vi "PCO_GetCameraDescription_Intensified.vi"(8 "error in (no error)":errorcluster {"code" format="%x"}, 11 "ph":u64) -> (0 "error out":errorcluster {"code" format="%x"}, 1 "strDescription":T1 {"dwFlagsIntensifiedDESC" format="%x"}, 2 "ErrorMessage":i32 format="%x", 3 "ph out":u64)   [LabVIEW 2020, in "SDK.lvlib" / "SpecialCommandsDicam.lvlib"]
doc: "<b>Description:</b>\nAny of the available sensor and camera specific description can be queried. With input parameter wType the returned description structure can be selected. PCO_DescriptionEx is a generic structure which has to be casted to/from the queried structure. The wSize parameter has to be filled with the correct value for the requested structure. This function was introduced due to the size limitation of the standard camera descriptor and the need for describing additional features.\n\n<b>Supported camera type:</b>\nAll cameras\n\n<b>Descriptor dependency:</b>\ndwGeneralCapsDESC1: ENHANCED_DESCRIPTOR_2"
uses:
  SpecialCommandsDicam.lvlib
  Structures.lvlib
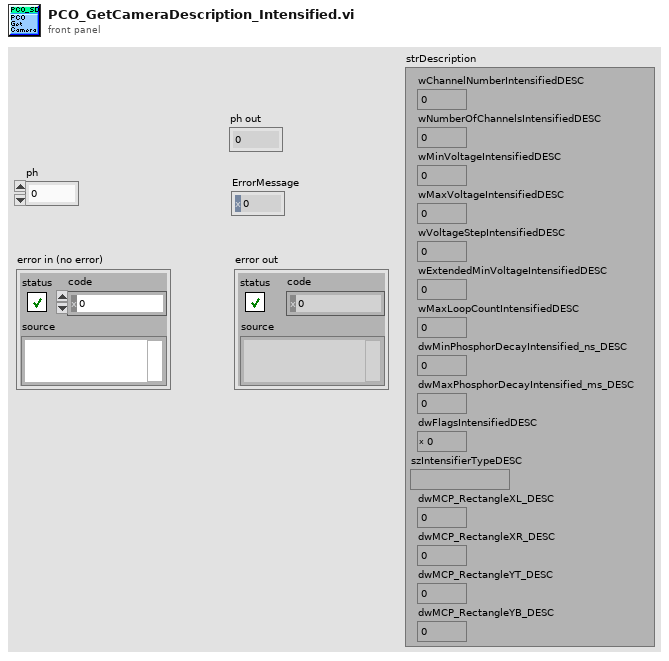
[diagram p1: front panel]
types:
  T1 = cluster{"wChannelNumberIntensifiedDESC":u16, "wNumberOfChannelsIntensifiedDESC":u16, "wMinVoltageIntensifiedDESC":u16, "wMaxVoltageIntensifiedDESC":u16, "wVoltageStepIntensifiedDESC":u16, "wExtendedMinVoltageIntensifiedDESC":u16, "wMaxLoopCountIntensifiedDESC":u16, "dwMinPhosphorDecayIntensified_ns_DESC":u32, "dwMaxPhosphorDecayIntensified_ms_DESC":u32, "dwFlagsIntensifiedDESC":u32, "szIntensifierTypeDESC":string, "dwMCP_RectangleXL_DESC":u32, "dwMCP_RectangleXR_DESC":u32, "dwMCP_RectangleYT_DESC":u32, "dwMCP_RectangleYB_DESC":u32}
  T2 = cluster{"wSize":u16, "wChannelNumberIntensifiedDESC":u16, "wNumberOfChannelsIntensifiedDESC":u16, "wMinVoltageIntensifiedDESC":u16, "wMaxVoltageIntensifiedDESC":u16, "wVoltageStepIntensifiedDESC":u16, "wExtendedMinVoltageIntensifiedDESC":u16, "wMaxLoopCountIntensifiedDESC":u16, "dwMinPhosphorDecayIntensified_ns_DESC":u32, "dwMaxPhosphorDecayIntensified_ms_DESC":u32, "dwFlagsIntensifiedDESC":u32, "szIntensifierTypeDESC":cluster{u8, u8, u8, u8, u8, u8, u8, u8, u8, u8, u8, u8, u8, u8, u8, u8, u8, u8, u8, u8, u8, u8, u8, u8}, "dwMCP_RectangleXL_DESC":u32, "dwMCP_RectangleXR_DESC":u32, "dwMCP_RectangleYT_DESC":u32, "dwMCP_RectangleYB_DESC":u32, "ZZdwDummy":cluster{u32, u32, u32, u32, u32, u32, u32, u32, u32, u32, u32, u32, u32, u32, u32, u32, u32, u32, u32, u32, u32, u32, u32}}
  T3 = cluster{u8, u8, u8, u8, u8, u8, u8, u8, u8, u8, u8, u8, u8, u8, u8, u8, u8, u8, u8, u8, u8, u8, u8, u8}
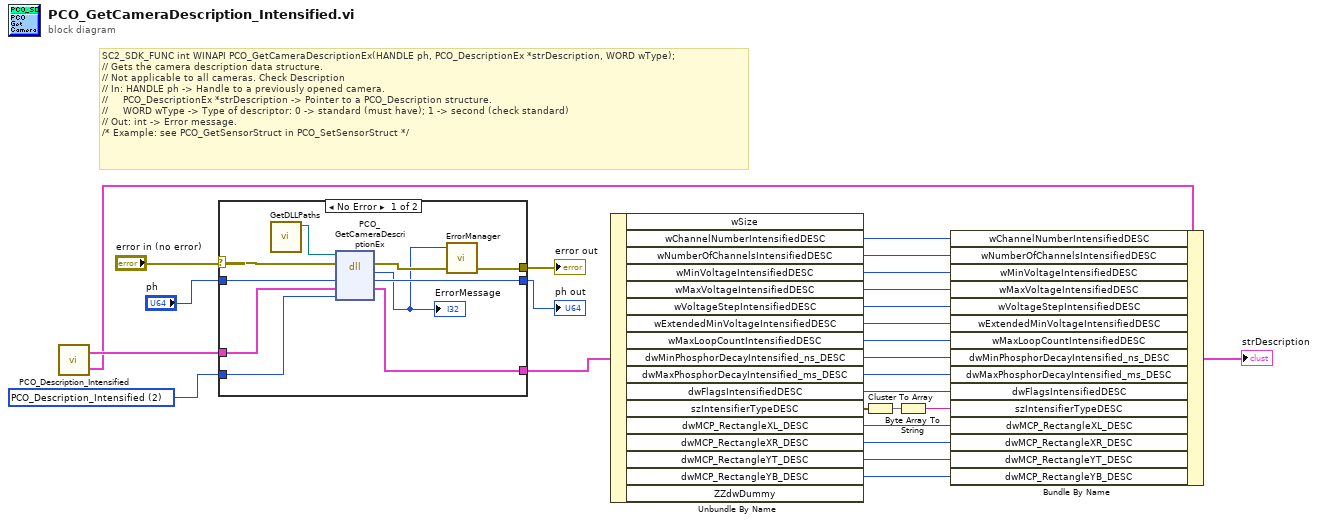
[diagram p0: block diagram]
diagram:
  w21 = u16 2 items=["PCO_Description", "PCO_Description2", "PCO_Description_Intensified"] ("wType")
  # "SC2_SDK_FUNC int WINAPI PCO_GetCameraDescriptionEx(HANDLE ph, PCO_DescriptionEx *strDescription, WORD wType);\n// Gets the camera description data structure.\n// Not applicable to all cameras. Check Description\n// In: HANDLE ph -> Handle to a previously opened camera.\n//     PCO_DescriptionEx *strDescription -> Pointer to a PCO_Description structure.\n//     WORD wType -> Type of descriptor: 0 -> standard (must have); 1 -> second (check standard)\n// Out: int -> Error message.\n/* Example: see PCO_GetSensorStruct in PCO_SetSensorStruct */"
  n1 = call "PCO_Description_Intensified.vi"() -> ("PCO_Description_Intensified"=w20:T1, "PCO_Description_Intensified_Raw"=w22:T2)  [unwired: 4 in, 2 out]
  n2 = case shown="No Error" "error in (no error)" {
    selector: "error in (no error)" -> [w35 w39]
    tunnel: "ph" -> [w36 w38]
    tunnel: w22 -> [w30 w37]
    tunnel: [w32 w39] -> w24
    tunnel: [w34 w38] -> w23
    tunnel: [w29 w37] -> w18
    tunnel: w21 -> [w28 _]
    frame No Error {
      n3 = call "GetDLLPaths.vi"() -> ("SC2_Cam_Path"=w27:path)  [unwired: 9 in, 2 out]
      n4 = dll-call lib="?" fn="PCO_GetCameraDescriptionEx"(path in=w27, error in=w35, "ph"=w36, "strDescription"=w30, "wType"=w28) -> (error out=w33:errorcluster, "return type"=w31:i32, "ph"=w34:u64, "strDescription"=w29:T2)  [unwired: 2 in, 1 out]
      "ErrorMessage" <- w31
      n5 = call "ErrorManager.vi"("error in (no error)"=w33, "error code"=w31) -> ("error out"=w32:errorcluster)  [unwired: 3 in]
    }
    frame Error {
    }
  }
  "error out" <- w24
  "ph out" <- w23
  n6 = Unbundle By Name(w18) -> ("wChannelNumberIntensifiedDESC"=w14:u16, "wNumberOfChannelsIntensifiedDESC"=w13:u16, "wMinVoltageIntensifiedDESC"=w12:u16, "wMaxVoltageIntensifiedDESC"=w11:u16, "wVoltageStepIntensifiedDESC"=w10:u16, "wExtendedMinVoltageIntensifiedDESC"=w9:u16, "wMaxLoopCountIntensifiedDESC"=w8:u16, "dwMinPhosphorDecayIntensified_ns_DESC"=w7:u32, "dwMaxPhosphorDecayIntensified_ms_DESC"=w6:u32, "dwFlagsIntensifiedDESC"=w5:u32, "szIntensifierTypeDESC"=w17:T3, "dwMCP_RectangleXL_DESC"=w4:u32, "dwMCP_RectangleXR_DESC"=w3:u32, "dwMCP_RectangleYT_DESC"=w2:u32, "dwMCP_RectangleYB_DESC"=w1:u32)  [unwired: 2 out]
  n7 = Cluster To Array(cluster=w17) -> (array=w16:u8[])
  n8 = Byte Array To String(unsigned byte array=w16) -> (string=w15:string)
  n9 = Bundle By Name(cluster=w20, "wChannelNumberIntensifiedDESC"=w14, "wNumberOfChannelsIntensifiedDESC"=w13, "wMinVoltageIntensifiedDESC"=w12, "wMaxVoltageIntensifiedDESC"=w11, "wVoltageStepIntensifiedDESC"=w10, "wExtendedMinVoltageIntensifiedDESC"=w9, "wMaxLoopCountIntensifiedDESC"=w8, "dwMinPhosphorDecayIntensified_ns_DESC"=w7, "dwMaxPhosphorDecayIntensified_ms_DESC"=w6, "dwFlagsIntensifiedDESC"=w5, "szIntensifierTypeDESC"=w15, "dwMCP_RectangleXL_DESC"=w4, "dwMCP_RectangleXR_DESC"=w3, "dwMCP_RectangleYT_DESC"=w2, "dwMCP_RectangleYB_DESC"=w1) -> (→"strDescription":T1)
